vi "G#Object_ExternalCreateProcess.vi"(0 "occurrence":refnum<k4>, 5 "error in (no error)":errorcluster) -> (19 "error out":errorcluster)   [LabVIEW 2017, in "G#Object.lvclass"]
doc: "This is an external create process that will create an own all objects. It is stopped when running the garbage collector."
uses:
  G#Object.lvclass
  utils/G#Object_Event.ctl
  utils/G#Object_EventType.ctl
  utils/G#Object_ObjectInfoType.ctl
  utils/G#Object_CreateMethod.ctl
  <vilib>/Utility/error.llb/Error Cluster From Error Code.vi
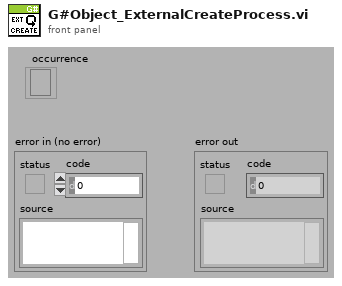
[diagram p1: front panel]
types:
  T1 = typedef "G#Object.lvclass/G#Object_Event.ctl" = cluster{"EventType":T2, "ObjectInfo":T3, "Ref":refnum<class "G#Object.lvclass">, "Time Stamp":timestamp, "LogText":string, "Parameters":variant[]}
  T2 = typedef "G#Object.lvclass/G#Object_EventType.ctl" = enum16{"Created new", "Looked up existing", "Deleted", "Forced delete", "Not deleted", "Garbage collected", "Cleared", "User", "Error", "External create object", "External create class attributes", "Created class attributes", "Run constructor", "Run constructor done", "Run open method", "Run open method done"}
  T3 = typedef "G#Object.lvclass/G#Object_ObjectInfoType.ctl" = cluster{"ObjectName":string, "ObjectID":u32, "Users":i32, "Counter":bool, "AttributeRefs":u32[], "FullClassName":string, "ClassName":string, "CreateMethod":T4, "GenericDestructorExists":bool, "Owner":string}
  T4 = typedef "G#Object.lvclass/G#Object_CreateMethod.ctl" = enum16{"Create", "Create or look up existing", "Look up existing"}
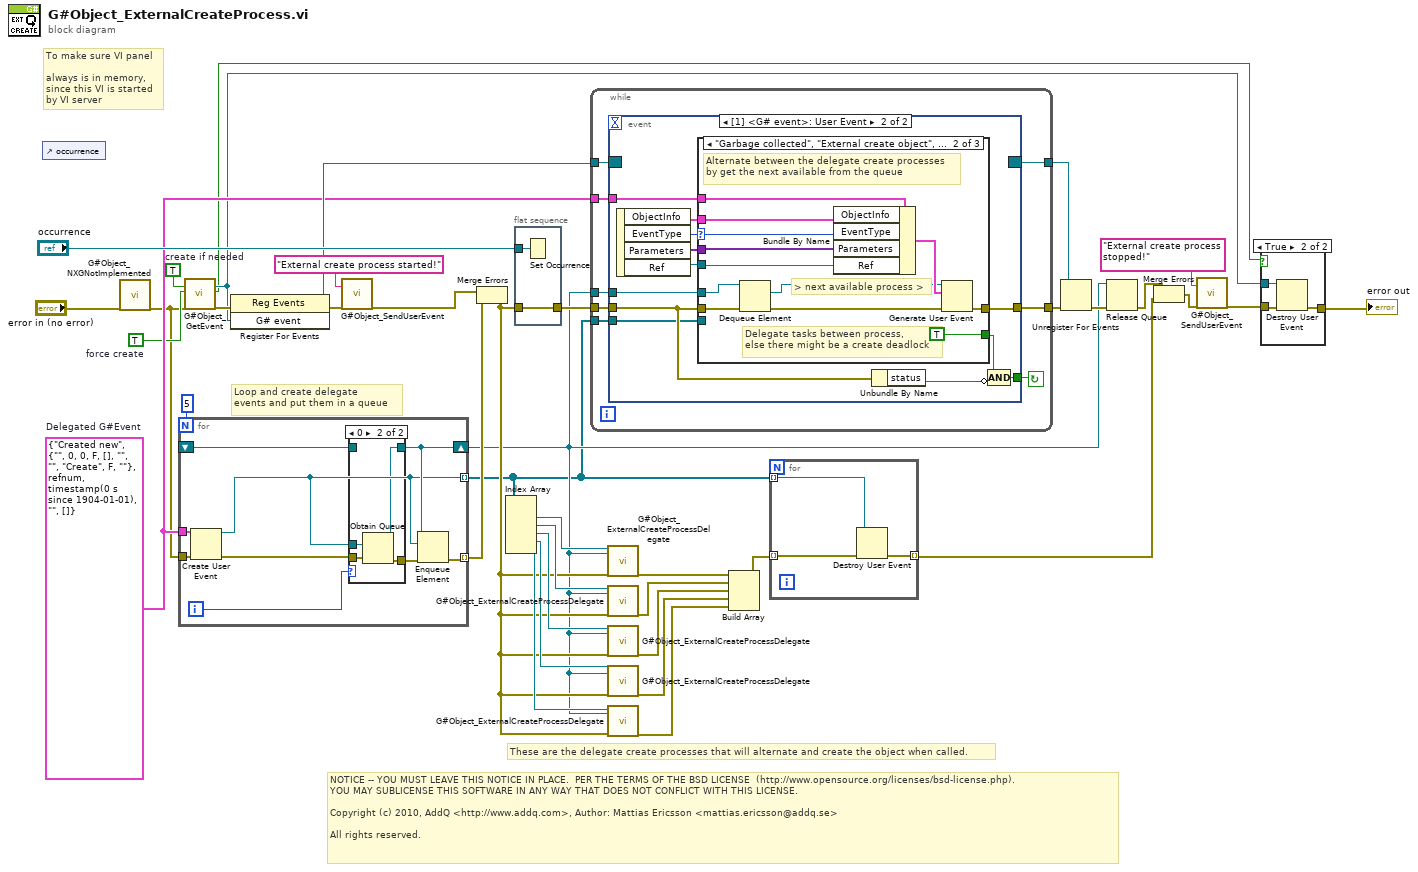
[diagram p0: block diagram]
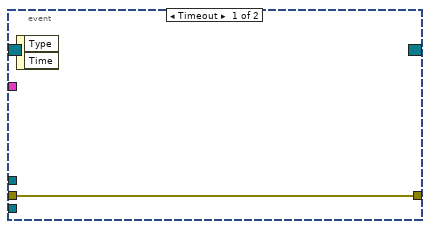
[diagram p4: hidden frame]
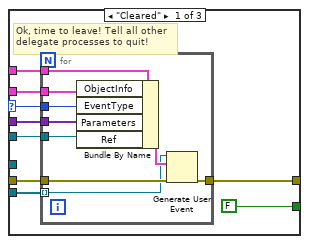
[diagram p5: hidden frame]
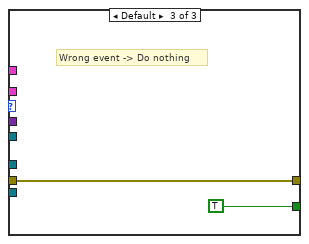
[diagram p6: hidden frame]
diagram:
  w5 = TRUE  # force create
  w31 = T1 {"EventType"=enum."Created new", "ObjectInfo"={"ObjectName"="", "ObjectID"=0, "Users"=0, "Counter"=FALSE, "AttributeRefs"=[], "FullClassName"="", "ClassName"="", "CreateMethod"=enum."Create", "GenericDestructorExists"=FALSE, "Owner"=""}, "Ref"=refnum, "Time Stamp"=timestamp(0 s since 1904-01-01), "LogText"="", "Parameters"=[]}  # Delegated G#Event
  w38 = TRUE  # create if needed
  # "Loop and create delegate\nevents and put them in a queue"
  # "These are the delegate create processes that will alternate and create the object when called."
  # "To make sure VI panel\n\nalways is in memory,\nsince this VI is started\nby VI server"
  # "NOTICE -- YOU MUST LEAVE THIS NOTICE IN PLACE.  PER THE TERMS OF THE BSD LICENSE  (http://www.opensource.org/licenses/bsd-license.php).\nYOU MAY SUBLICENSE THIS SOFTWARE IN ANY WAY THAT DOES NOT CONFLICT WITH THIS LICENSE.\n\nCopyright (c) 2010, AddQ <http://www.addq.com>, Author: Mattias Ericsson <mattias.ericsson@addq.se>\n\nAll rights reserved."
  n1 = control-ref of="occurrence"() -> ()  [unwired: 1 out]
  n2 = call "G#Object_NXGNotImplemented.vi"("error in"="error in (no error)") -> ("error out"=w2:errorcluster)  [unwired: 18 in]
  n3 = for {
    N: 5 -> [_]
    tunnel: w31 -> [w48]
    tunnel: w2 -> [w47]
    tunnel: [w42] -> w4 mode=indexing
    tunnel: [w41] -> w26 mode=indexing
    shift-right: [w43] -> w10
    shift-left: _ -> [w45]
    i -> [w46]
    n4 = Create User Event(user event datatype=w48, error in=w47) -> (user event=w42:refnum<user-event>, error out=w40:errorcluster)
    n5 = case shown="0" w46 {
      tunnel: w40 -> [w49 w54]
      tunnel: w42 -> [_ w53]
      tunnel: [w50 w52] -> w43
      tunnel: w45 -> [w50 _]
      tunnel: [w49 w51] -> w44
      frame Default {
      }
      frame 0 {
        n6 = Obtain Queue(element data type=w53, error in (no error)=w54) -> (queue out=w52:refnum<queue>, error out=w51:errorcluster)  [unwired: 3 in, 1 out]
      }
    }
    n7 = Enqueue Element(queue=w43, element=w42, error in (no error)=w44) -> (error out=w41:errorcluster)  [unwired: 1 in, 2 out]
  }
  n8 = call "G#Object_GetEvent.vi"("create if needed (T)"=w38, "force create (F)"=w5, "error in (no error)"=w2) -> ("G# event"=w7:refnum<user-event>, "created new"=w6:bool, "error out"=w37:errorcluster)  [unwired: 12 in, 2 out]
  n9 = register-events(error in=w37, w7) -> (reference out=w35:refnum<event-registration>, error out=w34:errorcluster)  [unwired: 1 in]
  n10 = call "G#Object_SendUserEvent.vi"("text"="External create process started!" ("Text"), "error in (no error)"=w34) -> ("error out"=w30:errorcluster)  [unwired: 16 in, 1 out]
  n11 = Merge Errors(w30, w26) -> (w15:errorcluster)
  n12 = Index Array(array=w4) -> (element #1=w20:refnum<user-event>, element #2=w19:refnum<user-event>, element #3=w18:refnum<user-event>, element #4=w17:refnum<user-event>, element #5=w16:refnum<user-event>)  [unwired: 5 in]
  n13 = flat-sequence {
    tunnel: "occurrence" -> [w56]
    tunnel: w15 -> [w55]
    tunnel: [w55] -> w14
    frame #0 {
      n14 = Set Occurrence(w56) -> ()
    }
  }
  n15 = while {
    tunnel: w14 -> [w64]
    tunnel: [w63] -> w32
    tunnel: w35 -> [w62]
    tunnel: [w61] -> w36
    tunnel: w31 -> [w59]
    tunnel: w10 -> [w58]
    tunnel: w4 -> [w57]
    stop <- w60 continue-if-true
    n16 = event shown="[1] <G# event>: User Event" {
      selector: w62 -> [_ _]
      dyn-events: [_ _] -> w61
      timeout: _ -> [_ _]
      tunnel: w64 -> [w65 w75]
      tunnel: [w65 w77] -> w63
      tunnel: [_ w72] -> w60
      tunnel: w59 -> [_ w69]
      tunnel: w58 -> [_ w68]
      tunnel: w57 -> [_ w67]
      event Timeout {
        n17 = event-data() -> ()  [unwired: 1 in, 2 out]
      }
      event User Event {
        n18 = event-data() -> ("ObjectInfo"=w70:T3, "EventType"=w76:T2, "Parameters"=w71:variant[], "Ref"=w66:refnum<class "G#Object.lvclass">)  [unwired: 1 in]
        n19 = case shown="\"Garbage collected\", \"External create object\", \"External create class attributes\", \"Run constructor\", \"Run open method\"" w76 {
          selector: w76 -> [w83 w103 _]
          tunnel: w75 -> [w82 w100 w108]
          tunnel: [w85 w106 w108] -> w77
          tunnel: [FALSE TRUE TRUE] -> w73
          tunnel: w71 -> [w79 w102 _]
          tunnel: w70 -> [w80 w104 _]
          tunnel: w69 -> [w84 w105 _]
          tunnel: w68 -> [_ w98 _]
          tunnel: w67 -> [w81 _ _]
          tunnel: w66 -> [w78 w96 _]
          frame "Cleared" {
            # "Ok, time to leave! Tell all other\ndelegate processes to quit!"
            n20 = for {
              tunnel: w82 -> [w95]
              tunnel: [w94] -> w85
              tunnel: w84 -> [w93]
              tunnel: w83 -> [w91]
              tunnel: w81 -> [w90] mode=indexing
              tunnel: w80 -> [w89]
              tunnel: w79 -> [w88]
              tunnel: w78 -> [w87]
              n21 = Bundle By Name(cluster=w93, "ObjectInfo"=w89, "EventType"=w91, "Parameters"=w88, "Ref"=w87) -> (w92:T1)
              n22 = Generate User Event(user event=w90, event data cluster=w92, error in=w95) -> (error out=w94:errorcluster)  [unwired: 1 in, 1 out]
            }
          }
          frame "Garbage collected", "External create object", "External create class attributes", "Run constructor", "Run open method" {
            # "> next available process >"
            # "Delegate tasks between process,\nelse there might be a create deadlock"
            # "Alternate between the delegate create processes\nby get the next available from the queue"
            n23 = Dequeue Element(queue=w98, error in (no error)=w100) -> (element=w97:refnum<user-event>, error out=w99:errorcluster)  [unwired: 1 in, 2 out]
            n24 = Bundle By Name(cluster=w105, "ObjectInfo"=w104, "EventType"=w103, "Parameters"=w102, "Ref"=w96) -> (w101:T1)
            n25 = Generate User Event(user event=w97, event data cluster=w101, error in=w99) -> (error out=w106:errorcluster)  [unwired: 1 in, 1 out]
          }
          frame Default {
            # "Wrong event -> Do nothing"
          }
        }
        n26 = Unbundle By Name(w75) -> ("status"=w74:bool)
        n27 = Compound Arithmetic op=AND(w73, invert w74) -> (w72:bool)
      }
    }
  }
  n28 = call "G#Object_ExternalCreateProcessDelegate.vi"("delegate event out"=w20, "event queue"=w10, "error in (no error)"=w15) -> ("error out"=w27:errorcluster)  [unwired: 16 in]
  n29 = call "G#Object_ExternalCreateProcessDelegate.vi"("delegate event out"=w19, "event queue"=w10, "error in (no error)"=w15) -> ("error out"=w25:errorcluster)  [unwired: 16 in]
  n30 = call "G#Object_ExternalCreateProcessDelegate.vi"("delegate event out"=w18, "event queue"=w10, "error in (no error)"=w15) -> ("error out"=w24:errorcluster)  [unwired: 16 in]
  n31 = call "G#Object_ExternalCreateProcessDelegate.vi"("delegate event out"=w17, "event queue"=w10, "error in (no error)"=w15) -> ("error out"=w23:errorcluster)  [unwired: 16 in]
  n32 = call "G#Object_ExternalCreateProcessDelegate.vi"("delegate event out"=w16, "event queue"=w10, "error in (no error)"=w15) -> ("error out"=w22:errorcluster)  [unwired: 16 in]
  n33 = Build Array(w27, w25, w24, w23, w22) -> (w21:errorcluster[])
  n34 = for {
    tunnel: [w112] -> w28 mode=indexing
    tunnel: w4 -> [w111] mode=indexing
    tunnel: w21 -> [w110] mode=indexing
    n35 = Destroy User Event(user event=w111, error in=w110) -> (error out=w112:errorcluster)
  }
  n36 = Unregister For Events(event registration refnum=w36, error in=w32) -> (error out=w13:errorcluster)
  n37 = Release Queue(queue=w10, error in (no error)=w13) -> (error out=w12:errorcluster)  [unwired: 1 in, 2 out]
  n38 = Merge Errors(w12, w28) -> (w11:errorcluster)
  n39 = call "G#Object_SendUserEvent.vi"("text"="External create process stopped!" ("Text"), "error in (no error)"=w11) -> ("error out"=w8:errorcluster)  [unwired: 16 in, 1 out]
  n40 = case shown="True" w6 {
    tunnel: w8 -> [w113 w116]
    tunnel: [w113 w115] -> w1
    tunnel: w7 -> [_ w114]
    frame False {
    }
    frame True {
      n41 = Destroy User Event(user event=w114, error in=w116) -> (error out=w115:errorcluster)
    }
  }
  "error out" <- w1
